vi "Counter - Count Edges (Continuous Clock).vi"() -> ()   [LabVIEW 2022 SP3]
doc: "This example demonstrates how to continuously read back the number of digital edges that have been counted by a counter input. It uses an external clock so that the samples of the count register occur at regular intervals. If you do not need deterministic sampling of the count register, refer instead to the Count Edges example which does not use an external clock.\n\nFor instructions on how to connect your signals to the DAQ device, refer to your device documentation."
uses:
  <vilib>/Utility/error.llb/DialogType.ctl
  <vilib>/DAQmx/read.llb/DAQmx Read (Counter 1D U32 1Chan NSamp).vi
  <vilib>/DAQmx/create/channels.llb/DAQmx Create Channel (CI-Count Edges).vi
  <vilib>/DAQmx/configure/timing.llb/DAQmx Timing (Sample Clock).vi
  <vilib>/DAQmx/miscellaneous.llb/DAQmx Fill In Error Info.vi
  <resource>/objmgr/daqmx.rc
panel:
  in  "Active Edge":i32(ring)=10280 items=["Rising"=10280, "Falling"=10171]
  in  "Trigger Type":T1(tab)
  in  "Edge":i32(ring)=10280 items=["Rising"=10280, "Falling"=10171]
  in  "Digital Trigger Source":tag
  in  "Pause When":i32(ring)=10192 items=["High"=10192, "Low"=10214]
  in  "Pause Trigger Source":tag
  in  "Count Reset Terminal":tag
  in  "Edge":i32(ring)=10280 items=["Rising"=10280, "Falling"=10171]
  out "Data":u32[](array[numeric])
  in  "Input Terminal":tag="PFI8"
  in  "Counter":tag="Dev1/ctr0"
  in  "Stop":bool
  in  "Samples per Loop":i32=100
  in  "Sample Rate":dbl=1000.0
  in  "Sample Clock Source":tag="PFI0"
  # "Channel Settings"
  # "Acquired Data"
  # "Timing Settings"
  # "Trigger Settings"
  # "To configure and use a trigger or the count reset you must have the necessary tab selected above.  Not all hardware supports the above options--refer to your device documentation for more info."
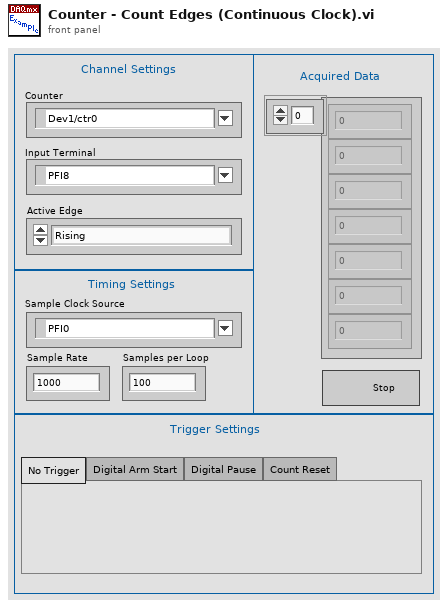
[diagram p1: front panel]
types:
  T1 = enum32{"No Trigger", "Digital Arm Start", "Digital Pause", "Count Reset"}
  T2 = typedef "DialogType.ctl" = u16
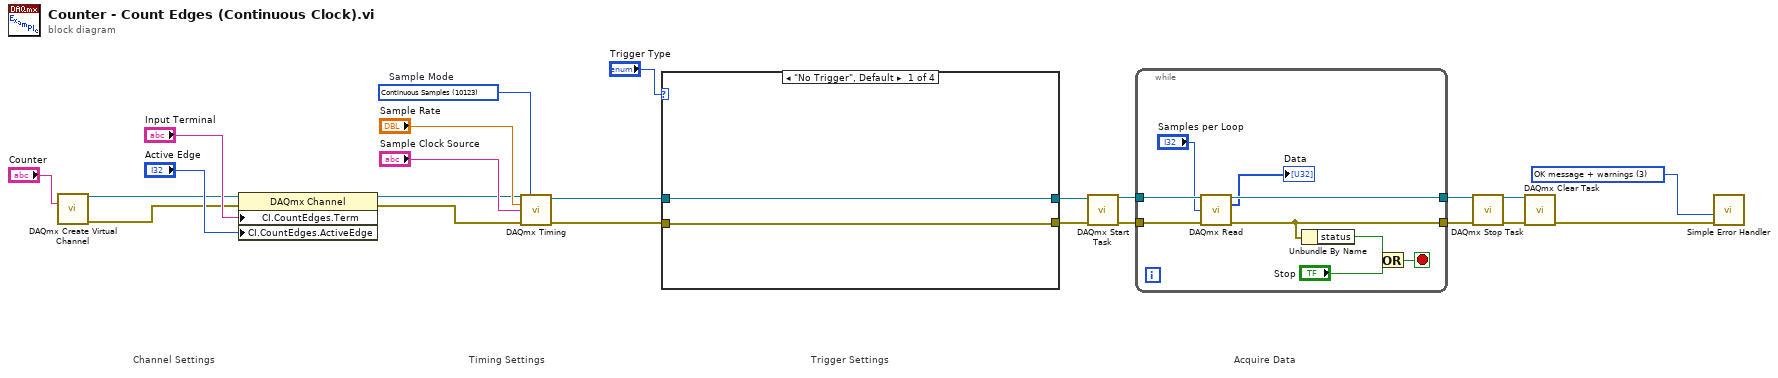
[diagram p0: block diagram]
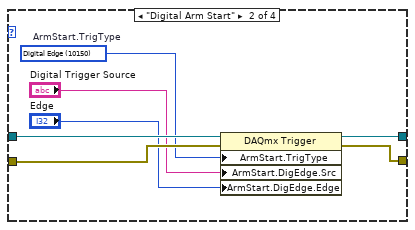
[diagram p2: hidden frame]
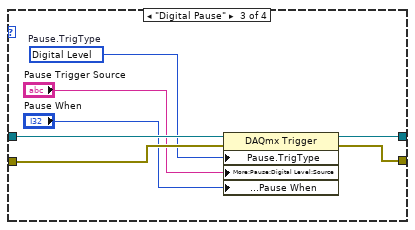
[diagram p3: hidden frame]
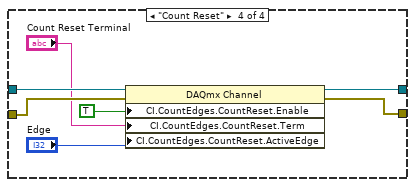
[diagram p4: hidden frame]
diagram:
  w1 = T2 3 items=["no dialog", "OK message", "continue or stop message", "OK message + warnings", "continue/stop + warnings"] ("type of dialog (OK msg:1)")
  w21 = 10123 items=["Finite Samples"=10178, "Continuous Samples"=10123, "Hardware Timed Single Point"=12522]  # Sample Mode
  # "Acquire Data"
  # "Trigger Settings"
  # "Timing Settings"
  # "Channel Settings"
  n1 = call-poly <vilib>:"DAQmx Create Virtual Channel.vi"("counter"="Counter") -> ("task out"=w14:refnum<k21>, "error out"=w11:errorcluster)  [unwired: 13 in]
  n2 = property class="DAQmx Channel"(reference=w14, error in=w11, "CI.CountEdges.Term"="Input Terminal", "CI.CountEdges.ActiveEdge"="Active Edge") -> (reference out=w13:refnum<k21>, error out=w12:errorcluster)
  n3 = call-poly <vilib>:"DAQmx Timing.vi"("task/channels in"=w13, "sample mode"=w21, "rate"="Sample Rate", "source"="Sample Clock Source", "error in"=w12) -> ("task out"=w7:refnum<k21>, "error out"=w6:errorcluster)  [unwired: 9 in]
  n4 = case shown="\"No Trigger\", Default" "Trigger Type" {
    tunnel: w7 -> [w25 w32 w39 w46]
    tunnel: w6 -> [w24 w29 w36 w43]
    tunnel: [w25 w31 w38 w45] -> w8
    tunnel: [w24 w30 w37 w44] -> w9
    frame "No Trigger", Default {
    }
    frame "Digital Arm Start" {
      w26 = 10150 items=["Digital Edge"=10150, "None"=10230]  # ArmStart.TrigType
      n5 = property class="DAQmx Trigger"(reference=w32, error in=w29, "ArmStart.TrigType"=w26, "ArmStart.DigEdge.Src"="Digital Trigger Source", "ArmStart.DigEdge.Edge"="Edge") -> (reference out=w31:refnum<k21>, error out=w30:errorcluster)
    }
    frame "Digital Pause" {
      w35 = 10152 items=["Analog Level"=10101, "Analog Window"=10103, "Digital Level"=10152, "Digital Pattern"=10398, "None"=10230]  # Pause.TrigType
      n6 = property class="DAQmx Trigger"(reference=w39, error in=w36, "Pause.TrigType"=w35, "More:Pause:Digital Level:Source"="Pause Trigger Source", "More:Pause:Digital Level:Pause When"="Pause When") -> (reference out=w38:refnum<k21>, error out=w37:errorcluster)
    }
    frame "Count Reset" {
      n7 = property class="DAQmx Channel"(reference=w46, error in=w43, "CI.CountEdges.CountReset.Enable"=TRUE, "CI.CountEdges.CountReset.Term"="Count Reset Terminal", "CI.CountEdges.CountReset.ActiveEdge"="Edge") -> (reference out=w45:refnum<k21>, error out=w44:errorcluster)
    }
  }
  n8 = call <vilib>:"DAQmx Start Task.vi"("task/channels in"=w8, "error in"=w9) -> ("task out"=w20:refnum<k21>, "error out"=w19:errorcluster)  [unwired: 12 in]
  n9 = while {
    tunnel: w20 -> [w55]
    tunnel: w19 -> [w54]
    tunnel: [w51] -> w4
    tunnel: [w52] -> w5
    stop <- w53 stop-if-true
    n10 = call-poly <vilib>:"DAQmx Read.vi"("task/channels in"=w55, "number of samples per channel"="Samples per Loop", "error in"=w54) -> ("task out"=w52:refnum<k21>, "data"=→"Data":u32[], "error out"=w51:errorcluster)  [unwired: 10 in]
    n11 = Unbundle By Name(w51) -> ("status"=w50:bool)
    n12 = Or(x=w50, y="Stop") -> (x .or. y?=w53:bool)
  }
  n13 = call <vilib>:"DAQmx Stop Task.vi"("task/channels in"=w5, "error in"=w4) -> ("task out"=w2:refnum<k21>, "error out"=w3:errorcluster)  [unwired: 12 in]
  n14 = call <vilib>:"DAQmx Clear Task.vi"("task in"=w2, "error in"=w3) -> ("error out"=w18:errorcluster)  [unwired: 13 in]
  n15 = call <vilib>:"Simple Error Handler.vi"("type of dialog (OK msg:1)"=w1, "error in (no error)"=w18) -> ()  [unwired: 3 in, 5 out]
